vi "Server Thread Handle Message (Targets Message).vi"(3 "error in":errorcluster, 4 "Targets Message":T3={"capturedAgoMs"=0, "targets"=[{"x"=0.0, "y"=0.0, "z"=0.0, "theta"=0.0}]}, 5 "Timestamp":dbl format="%#_13g", 6 "Server Thread":T1) -> (0 "error out":errorcluster, 1 "Targets Update":T2, 2 "Server Thread":T1)   [LabVIEW 2016]
uses:
  Messages/Targets/Targets Message.ctl
  Messages/Targets/Targets Info.ctl
  Messages/Targets/Targets Update.ctl
  Server Thread.ctl
  Messages/Heartbeat/Heartbeat Message to JSON.vi
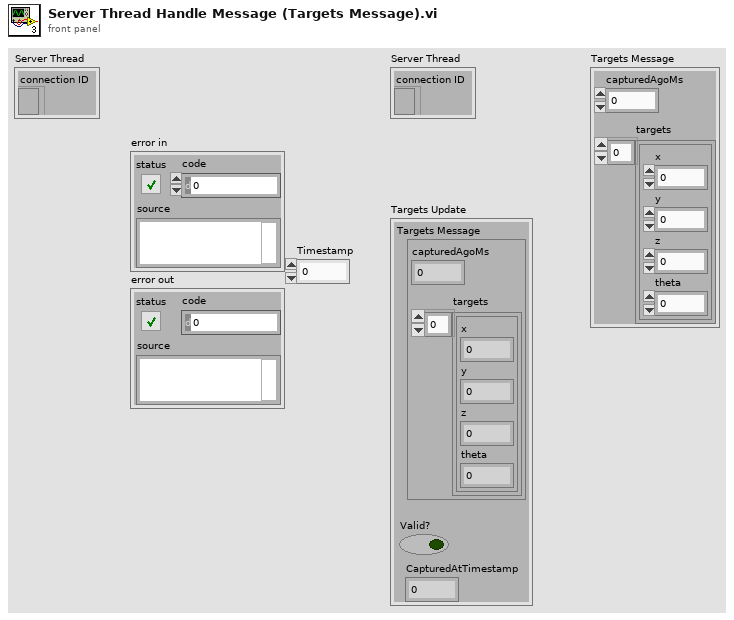
[diagram p1: front panel]
types:
  T1 = typedef "Server Thread.ctl" = cluster{"connection ID":refnum<k5>}
  T2 = typedef "Targets Update.ctl" = cluster{"Valid?":bool, "CapturedAtTimestamp":dbl, "Targets Message":T3}
  T3 = typedef "Targets Message.ctl" = cluster{"capturedAgoMs":i32, "targets":T4[]}
  T4 = typedef "Targets Info.ctl" = cluster{"x":dbl, "y":dbl, "z":dbl, "theta":dbl}
  T5 = typedef "Heartbeat Message.ctl" = cluster{"type":string, "message":string}
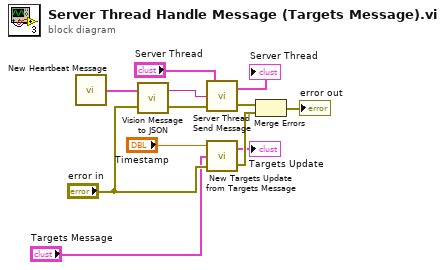
[diagram p0: block diagram]
diagram:
  n1 = call "New Heartbeat Message.vi"() -> ("Heartbeat Message"=w11:T5)
  n2 = call-poly "Vision Message to JSON.vi"("error in"="error in", "Heartbeat Message"=w11) -> ("error out"=w8:errorcluster, "JSON string"=w9:string)
  n3 = call "Server Thread Send Message.vi"("error in"=w8, "JSON string"=w9, "Server Thread"="Server Thread") -> ("error out"=w6:errorcluster, "Server Thread"=→"Server Thread":T1)
  n4 = call "New Targets Update from Targets Message.vi"("error in"="error in", "Targets Message"="Targets Message", "Current Time (ms)"="Timestamp") -> ("error out"=w5:errorcluster, "Targets Update"=→"Targets Update":T2)
  n5 = Merge Errors(w6, w5) -> (→"error out":errorcluster)
